vi "UDP3READ.vi"(0 "Frequency, in Hz":dbl) -> ()   [LabVIEW 2009]
doc: "Reads a UDP stream over channel 1338 (which should be comeing from UDP3LOOP.vi) which sends a flattened variant of the strict type def UDP3.ctl. This function restores this flattened string to the original shape (that of UDP3.ctl) and then passes it to the global variable (global on the rt processor anyway) UDP3rtglob.vi which can be read by outside functions. It's loop can be stopped by setting UDP3rtglob.vi.stop to true, in the same way it's sister function UDP3LOOP.vi is stopped using UDP3GLOB.vi.stop. Frequency is set via an input, and is implemented via quantized wait for ms multiple. The division is preformed only once."
uses:
  UDP 3.ctl
  UDP3rtglob.vi
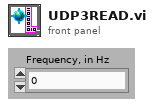
[diagram p1: front panel]
types:
  T1 = typedef "UDP 3.ctl" = cluster{"GPS":cluster{"Lat":dbl, "Longe":dbl}, "INS":cluster{"Compass":dbl, "Altitude":dbl, "Lat":dbl, "Longe":dbl}}
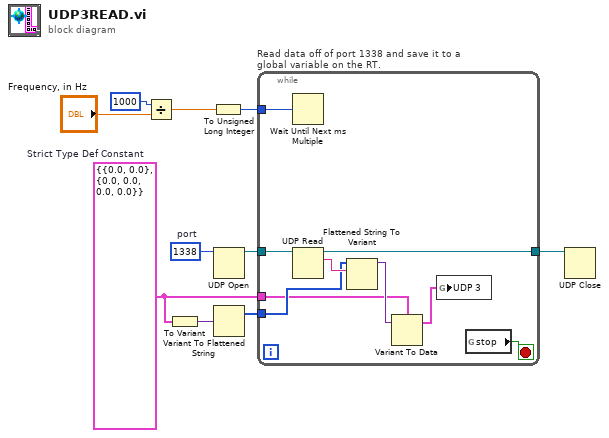
[diagram p0: block diagram]
diagram:
  w5 = T1 {"GPS"={"Lat"=0.0, "Longe"=0.0}, "INS"={"Compass"=0.0, "Altitude"=0.0, "Lat"=0.0, "Longe"=0.0}}  # Strict Type Def Constant
  w8 = u16 1338  # port
  n1 = Divide(x=1000, y="Frequency, in Hz") -> (x/y=w2:dbl)
  n2 = To Variant(anything=w5) -> (Variant=w7:variant)
  n3 = To Unsigned Long Integer(number=w2) -> (unsigned 32bit integer=w1:u32)
  n4 = UDP Open(11:w8) -> (port=w9:refnum<k16>)  [unwired: 4 in, 2 out]
  n5 = Variant To Flattened String(Variant=w7) -> (1:w6:i16[])  [unwired: 1 out]
  n6 = while "Read data off of port 1338 and save it to a global variable on the RT." {
    tunnel: [w19] -> w10
    tunnel: w9 -> [w18]
    tunnel: w6 -> [w15]
    tunnel: w5 -> [w14]
    tunnel: w1 -> [w11]
    stop <- w12 stop-if-true
    n7 = Wait Until Next ms Multiple(millisecond multiple=w11) -> ()  [unwired: 1 out]
    n8 = UDP Read(connection ID=w18) -> (data out=w17:string, 3:w19:refnum<k16>)  [unwired: 3 in, 3 out]
    n9 = Flattened String To Variant(6:w17, 7:w15) -> (3:w16:variant)  [unwired: 1 in, 1 out]
    n10 = Variant To Data(Variant=w16, type=w14) -> (data=w13:T1)  [unwired: 1 in, 1 out]
    n11 = global write "UDP3rtglob.vi" "UDP 3"(w13) -> ()
    n12 = global read "UDP3rtglob.vi" "stop"() -> (w12:bool)
  }
  n13 = UDP Close(connection ID=w10) -> ()  [unwired: 1 in, 2 out]
